vi "Get NumJoints.vi"(8 "error in (no error)":errorcluster) -> (0 "error out":errorcluster, 3 "num_joints":i32)   [LabVIEW 2013, in "ikfast_labview.lvlib"]
doc: "IKFAST_API int GetNumJoints();"
uses:
  ikfast_labview.lvlib
  ikfast_labview.dll
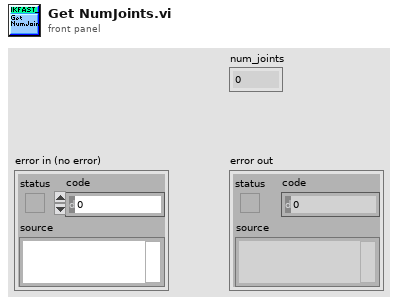
[diagram p1: front panel]
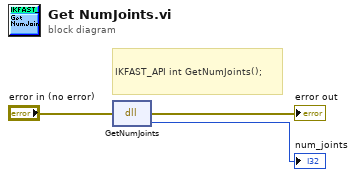
[diagram p0: block diagram]
diagram:
  # "IKFAST_API int GetNumJoints();"
  n1 = dll-call lib="C:/Users/fsuarez/git/ikfast_labview/user.lib/ikfast_labview/ikfast_labview.*" fn="GetNumJoints"(error in="error in (no error)") -> (error out=→"error out":errorcluster, →"num_joints":i32)  [unwired: 2 in, 1 out]
